vi "Historian.vi"(4 "Time of Completion":timestamp, 6 "Initial Time Stamp":timestamp, 7 "Initial Value":dbl, 8 "error in (no error)":errorcluster, 9 "Sampling Rates":dbl[](array[numeric]), 10 "setpoint profile":cluster{"time (s)":dbl, "setpoint":dbl}[](array[cluster]), 11 "Process_REF":string="Temperature") -> (0 "error out":errorcluster, 2 "Reports":T1(array[cluster]))   [LabVIEW 2018]
panel:
  out "Compare B":timestamp
  out "Compare A":timestamp
  out "Time of Now":timestamp
  out "Current Stage":dbl format="%_6g"
  out "Samples Taken":dbl
  out "Finished":bool
  in  "ManualAbort":bool
  out "ABORT":bool
  out "PV":dbl
  out "TIME":dbl format="%_6g"
  out "Take Sample":bool
  out "Time of Last Sample":timestamp
  out "Stage Sample Frequency":dbl
  out "Time of Next Sample":timestamp
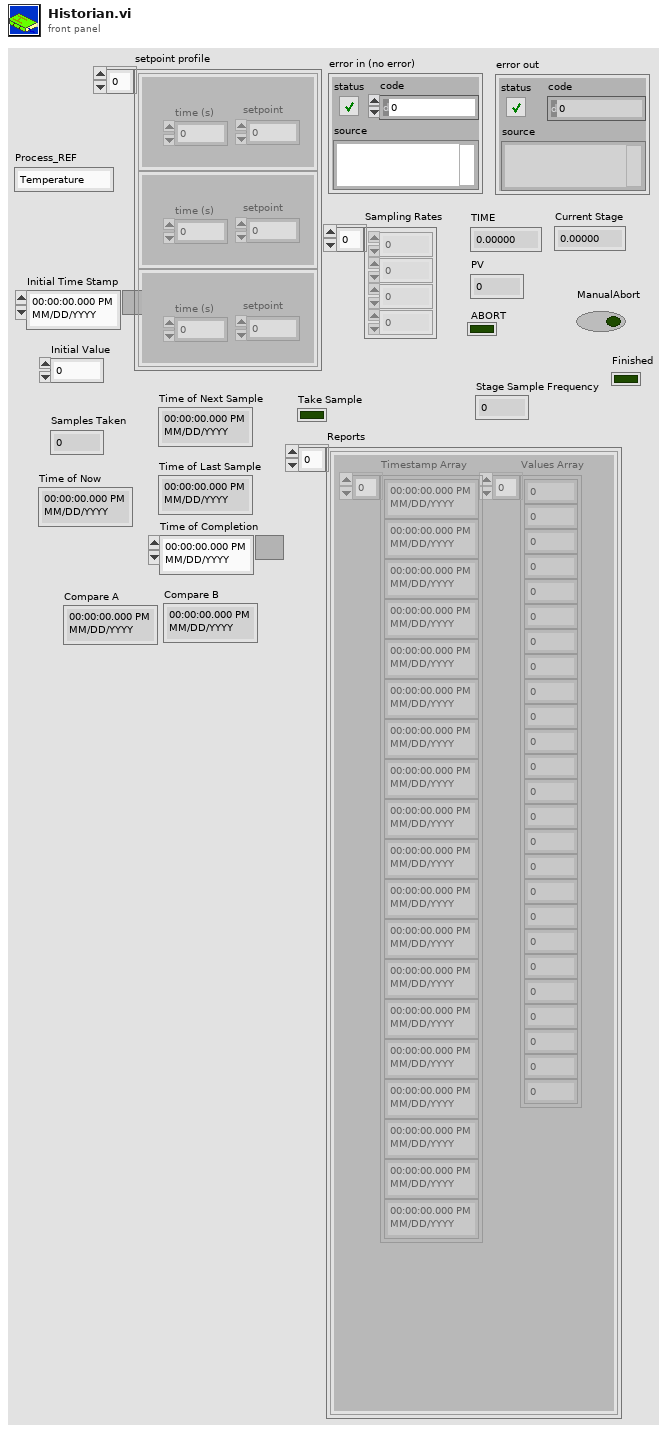
[diagram p1: front panel]
types:
  T1 = cluster{"Values Array":dbl[], "Timestamp Array":timestamp[]}[]
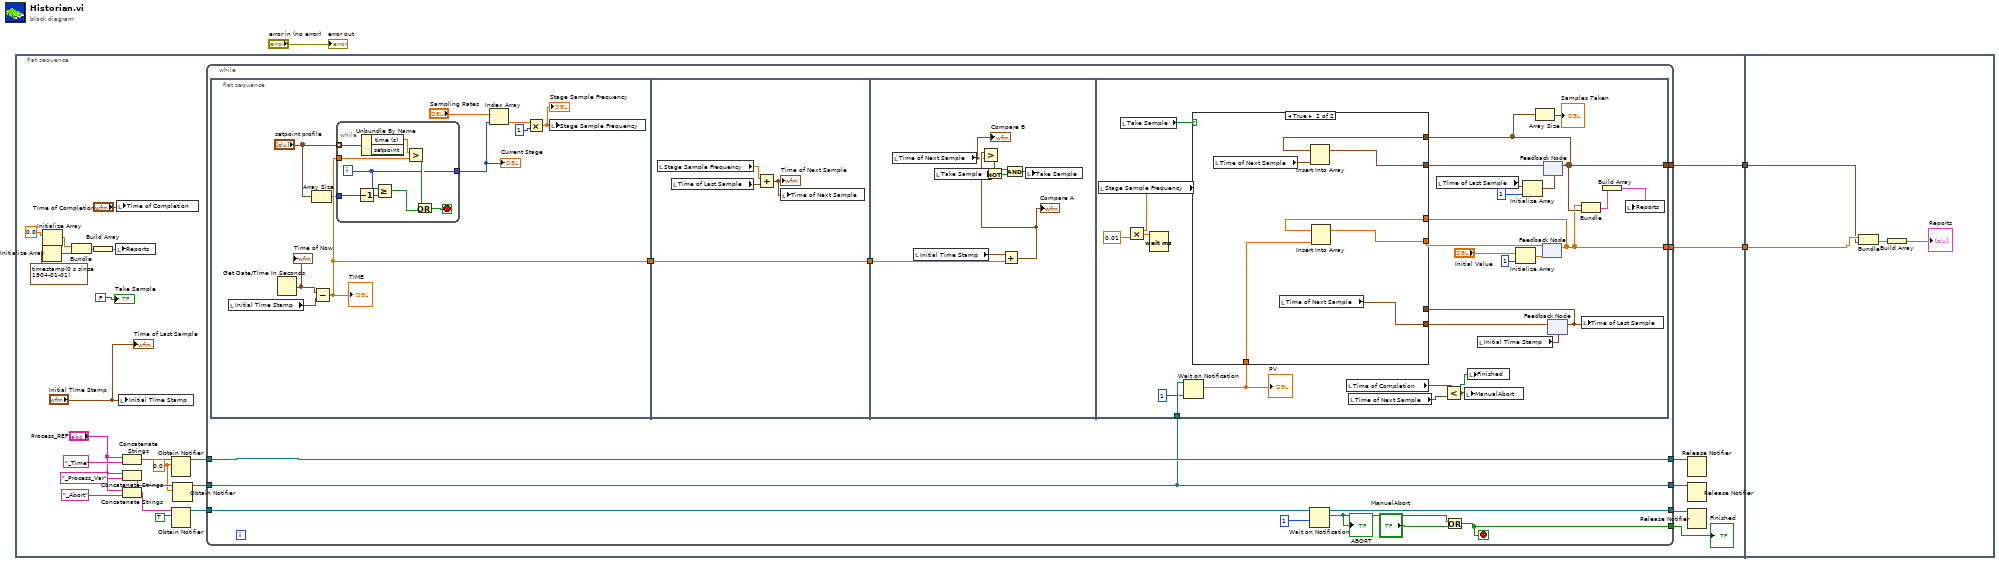
[diagram p0: block diagram]
diagram:
  n1 = flat-sequence {
    tunnel: [w26] -> w2
    tunnel: [w25] -> w1
    tunnel: w2 -> [w111]
    tunnel: w1 -> [w110]
    frame #0 {
      w17 = 0.0
      n2 = Initialize Array(timestamp(0 s since 1904-01-01)) -> (w6:timestamp[])  [unwired: 1 in]
      n3 = Initialize Array(0.0) -> (w5:dbl[])  [unwired: 1 in]
      n4 = Bundle(w5, w6) -> (w10:cluster{dbl[], timestamp[]})  [unwired: 1 in]
      n5 = Build Array(w10) -> (w8:cluster{dbl[], timestamp[]}[])
      n6 = local write "Reports"(w8) -> ()
      n7 = local write "Time of Completion"("Time of Completion") -> ()
      n8 = local write "Initial Time Stamp"("Initial Time Stamp") -> ()
      n9 = Concatenate Strings("Process_REF", "_Time") -> (w18:string)
      n10 = Concatenate Strings("Process_REF", "_Process_Var") -> (w20:string)
      n11 = Concatenate Strings("Process_REF", "_Abort") -> (w24:string)
      n12 = Obtain Notifier(name (unnamed)=w18, notification data type=w17) -> (notifier out=w19:refnum<notifier>)  [unwired: 2 in, 2 out]
      n13 = Obtain Notifier(name (unnamed)=w24, notification data type=TRUE) -> (notifier out=w23:refnum<notifier>)  [unwired: 2 in, 2 out]
      n14 = Obtain Notifier(name (unnamed)=w20, notification data type=w17) -> (notifier out=w21:refnum<notifier>)  [unwired: 2 in, 2 out]
      n15 = while {
        tunnel: [w38] -> w14
        tunnel: w19 -> [w38]
        tunnel: [w33] -> w15
        tunnel: w21 -> [w33]
        tunnel: [w39] -> w16
        tunnel: w23 -> [w40]
        tunnel: [w42] -> w26
        tunnel: [w41] -> w25
        tunnel: [w34] -> w13
        stop <- w34 stop-if-true
        n16 = flat-sequence {
          tunnel: [w48] -> w32
          tunnel: w32 -> [w65]
          tunnel: [w65] -> w31
          tunnel: w31 -> [w72]
          tunnel: [w79] -> w42
          tunnel: [w80] -> w41
          tunnel: w33 -> [w88]
          frame #0 {
            n17 = local read "Initial Time Stamp"() -> (w46:timestamp)
            n18 = Get Date/Time In Seconds() -> (seconds since 1Jan1904=w43:timestamp)
            "Time of Now" <- w43
            n19 = Array Size(array="setpoint profile") -> (size(s)=w44:i32)
            n20 = Subtract(x=w43, y=w46) -> (x-y=w48:dbl)
            "TIME" <- w48
            n21 = while {
              tunnel: "setpoint profile" -> [w61] mode=indexing
              tunnel: w48 -> [w60]
              tunnel: [w56] -> w47
              tunnel: w44 -> [w53]
              i -> [w56]
              stop <- w58 stop-if-true
              n22 = Decrement(x=w53) -> (x-1=w54:i32)
              n23 = Unbundle By Name(w61) -> ("time (s)"=w59:dbl)  [unwired: 1 out]
              n24 = Greater Or Equal?(x=w56, y=w54) -> (x >= y?=w55:bool)
              n25 = Greater?(x=w59, y=w60) -> (0:w57:bool)
              n26 = Or(x=w57, y=w55) -> (x .or. y?=w58:bool)
            }
            "Current Stage" <- w47
            n27 = Index Array(array="Sampling Rates", index=w47) -> (element=w50:dbl)
            n28 = Multiply(x=w50, y=1) -> (x*y=w49:dbl)
            "Stage Sample Frequency" <- w49
            n29 = local write "Stage Sample Frequency"(w49) -> ()
          }
          frame #1 {
            n30 = local read "Stage Sample Frequency"() -> (w64:dbl)
            n31 = local read "Time of Last Sample"() -> (w63:timestamp)
            n32 = Add(x=w64, y=w63) -> (x+y=w62:timestamp)
            "Time of Next Sample" <- w62
            n33 = local write "Time of Next Sample"(w62) -> ()
          }
          frame #2 {
            n34 = local read "Time of Next Sample"() -> (w70:timestamp)
            "Compare B" <- w70
            n35 = local read "Initial Time Stamp"() -> (w73:timestamp)
            n36 = local read "Take Sample"() -> (w69:bool)
            n37 = Not(x=w69) -> (.not. x?=w67:bool)
            n38 = Add(x=w73, y=w72) -> (x+y=w71:timestamp)
            "Compare A" <- w71
            n39 = Greater?(x=w71, y=w70) -> (0:w66:bool)
            n40 = And(x=w66, y=w67) -> (x .and. y?=w68:bool)
            n41 = local write "Take Sample"(w68) -> ()
          }
          frame #3 {
            n42 = local read "Stage Sample Frequency"() -> (w75:dbl)
            n43 = local read "Take Sample"() -> (w98:bool)
            n44 = Multiply(x=w75, y=0.01) -> (x*y=w74:dbl)
            n45 = Wait (ms)(milliseconds to wait=w74) -> ()  [unwired: 1 out]
            n46 = Wait on Notification(notifier=w88, timeout in ms (-1)=1) -> (notification=w78:dbl)  [unwired: 2 in, 3 out]
            "PV" <- w78
            n47 = local read "Time of Completion"() -> (w77:timestamp)
            n48 = local read "Time of Next Sample"() -> (w86:timestamp)
            n49 = local read "Time of Last Sample"() -> (w96:timestamp)
            n50 = Less?(x=w77, y=w86) -> (x < y?=w85:bool)
            n51 = local write "ManualAbort"(w85) -> ()
            n52 = local write "Finished"(w85) -> ()
            n53 = local read "Initial Time Stamp"() -> (w87:timestamp)
            n54 = Initialize Array("Initial Value", 1) -> (w95:dbl[])
            n55 = Initialize Array(w96, 1) -> (w94:timestamp[])
            n56 = feedback #1(w95) -> (w79:dbl[])
            n57 = feedback #2(w94) -> (w80:timestamp[])
            n58 = Array Size(array=w80) -> (size(s)=→"Samples Taken":i32)
            n59 = feedback #3(w87) -> (w97:timestamp)
            n60 = case shown="True" w98 {
              tunnel: w80 -> [w102 w109]
              tunnel: w79 -> [w101 w108]
              tunnel: w97 -> [w100 _]
              tunnel: [w102 w103] -> w90
              tunnel: [w101 w107] -> w91
              tunnel: [w100 w106] -> w89
              tunnel: w78 -> [_ w104]
              frame False {
              }
              frame True {
                n61 = local read "Time of Next Sample"() -> (w105:timestamp)
                n62 = local read "Time of Next Sample"() -> (w106:timestamp)
                n63 = Insert Into Array(array=w109, new element=w105) -> (w103:timestamp[])  [unwired: 1 in]
                n64 = Insert Into Array(array=w108, new element=w104) -> (w107:dbl[])  [unwired: 1 in]
              }
            }
            n65 = feedback-in #1(w91) -> ()
            n66 = feedback-in #2(w90) -> ()
            n67 = feedback-in #3(w89) -> ()
            n68 = Bundle(w79, w80) -> (w82:cluster{dbl[], timestamp[]})  [unwired: 1 in]
            n69 = local write "Time of Last Sample"(w97) -> ()
            n70 = Build Array(w82) -> (w81:cluster{dbl[], timestamp[]}[])
            n71 = local write "Reports"(w81) -> ()
          }
        }
        n72 = Wait on Notification(notifier=w40, timeout in ms (-1)=1) -> (notifier out=w39:refnum<notifier>, notification=w37:bool)  [unwired: 2 in, 2 out]
        "ABORT" <- w37
        n73 = Or(x=w37, y="ManualAbort") -> (x .or. y?=w34:bool)
      }
      "Finished" <- w13
      n74 = Release Notifier(notifier=w14) -> ()  [unwired: 2 in, 3 out]
      n75 = Release Notifier(notifier=w15) -> ()  [unwired: 2 in, 3 out]
      n76 = Release Notifier(notifier=w16) -> ()  [unwired: 2 in, 3 out]
      "Time of Last Sample" <- "Initial Time Stamp"
      "Take Sample" <- FALSE
    }
    frame #1 {
      n77 = Bundle(w111, w110) -> (w113:cluster{dbl[], timestamp[]})  [unwired: 1 in]
      n78 = Build Array(w113) -> (→"Reports":cluster{dbl[], timestamp[]}[])
    }
  }
  "error out" <- "error in (no error)"
